vi "AssertsAlmostEqual.vi"(11 "error in (no error)":errorcluster) -> (15 "error out":errorcluster)   [LabVIEW 2016, in "DronaTest.lvlib"]
uses:
  APIs/Assert/AssertControlValue/AlmostEqual.vi
  <vilib>/addons/_JKI Toolkits/Caraya/classes/Assert/Assert Not Error.vi
  <vilib>/addons/_JKI Toolkits/Caraya/classes/Assert/Assert Error.vi
  DronaTest.lvlib
  <vilib>/addons/_JKI Toolkits/Caraya/classes/Test/Test.lvclass
  Drona.lvlib
  <vilib>/addons/_JKI Toolkits/Caraya/classes/Assert/Assert.lvclass
  APIs/Assert/AssertControlValue/AssertControlValue.lvlib
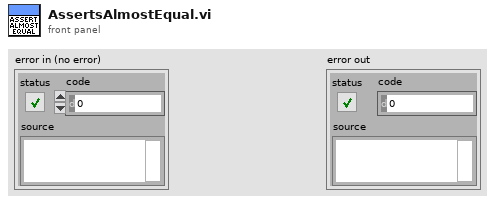
[diagram p1: front panel]
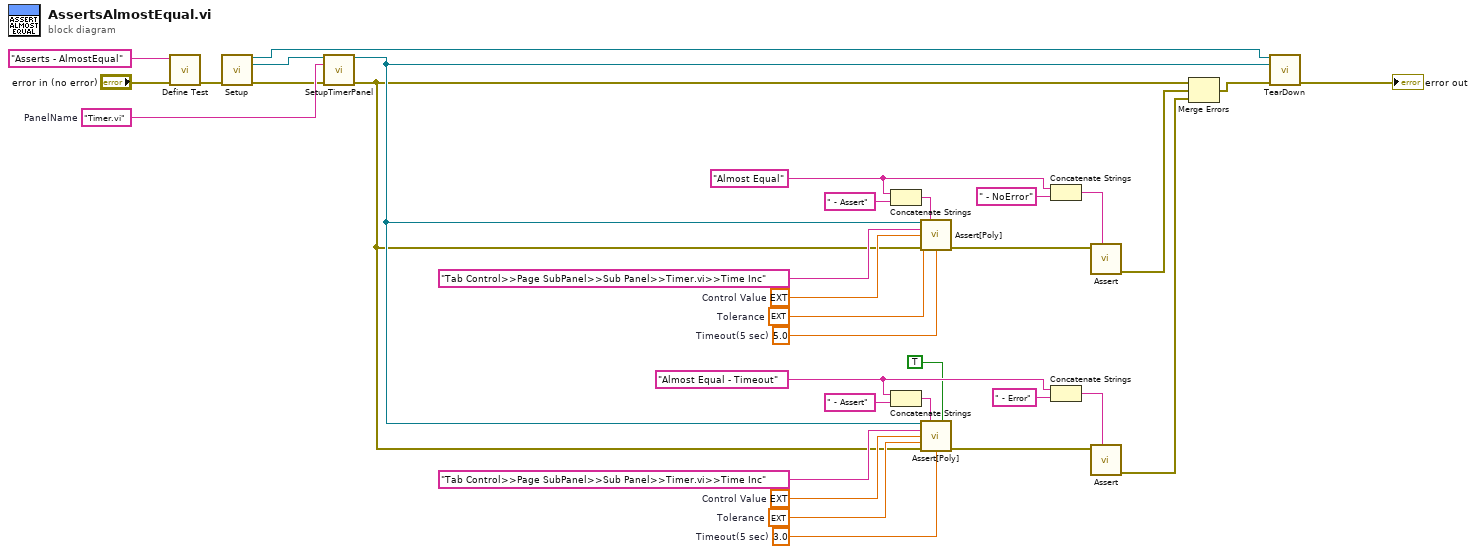
[diagram p0: block diagram]
diagram:
  w5 = "Timer.vi"  # PanelName
  w10 = ext 0.5  # Tolerance
  w11 = ext 0.5  # Tolerance
  w21 = 3.0  # Timeout(5 sec)
  w20 = ext 5.0  # Control Value
  w19 = "Almost Equal - Timeout" ("string")
  w22 = 5.0  # Timeout(5 sec)
  w23 = ext 5.0  # Control Value
  w24 = "Almost Equal" ("string")
  n1 = call <vilib>:"Define Test.vi"("error in (no error)"="error in (no error)", "Label (VI Title)"="Asserts - AlmostEqual") -> ("error out"=w9:errorcluster)  [unwired: 9 in]
  n2 = call "Setup.vi"("error in (no error)"=w9) -> ("Application Ref"=w6:refnum<vi>, "VI out"=w3:refnum<vi>, "error out"=w4:errorcluster)  [unwired: 12 in]
  n3 = call "SetupTimerPanel.vi"("VI in"=w3, "Panel Name"=w5, "error in (no error)"=w4) -> ("VI out"=w2:refnum<vi>, "error out"=w1:errorcluster)  [unwired: 11 in]
  n4 = Concatenate Strings(w24, " - Assert" ("string")) -> (w26:string)
  n5 = Concatenate Strings(w19, " - Assert" ("string")) -> (w17:string)
  n6 = call-poly "Assert[Poly].vi"("VI Reference In"=w2, "Test Label"=w26, "Control Path"="Tab Control>>Page SubPanel>>Sub Panel>>Timer.vi>>Time Inc", "Control Value"=w23, "Tolerance"=w11, "Error In"=w1, "Timeout(5 sec)"=w22) -> ("Error Out"=w27:errorcluster)  [unwired: 7 in, 1 out]
  n7 = call-poly "Assert[Poly].vi"("VI Reference In"=w2, "Test Label"=w17, "Assert Only? (F)"=TRUE, "Control Path"="Tab Control>>Page SubPanel>>Sub Panel>>Timer.vi>>Time Inc", "Control Value"=w20, "Tolerance"=w10, "Error In"=w1, "Timeout(5 sec)"=w21) -> ("Error Out"=w16:errorcluster)  [unwired: 6 in, 1 out]
  n8 = Concatenate Strings(w24, " - NoError" ("string")) -> (w25:string)
  n9 = Concatenate Strings(w19, " - Error" ("string")) -> (w18:string)
  n10 = call-poly <vilib>:"Assert.vi"("Label"=w25, "Not Error?"=w27) -> ("error out"=w34:errorcluster)  [unwired: 9 in]
  n11 = call-poly <vilib>:"Assert.vi"("Label"=w18, "Error?"=w16) -> ("error out"=w31:errorcluster)  [unwired: 9 in]
  n12 = Merge Errors(w1, w34, w31) -> (w8:errorcluster)
  n13 = call "TearDown.vi"("Application Ref"=w6, "VI in"=w2, "error in (no error)"=w8) -> ("error out"=→"error out":errorcluster)  [unwired: 12 in]
